vi "Teleop.vi"(10 "Match Info":T1={"Autonomous Elapsed Seconds"=0.0, "TeleOp Elapsed Seconds"=78.62, "Disabled Elapsed Seconds"=2.155, "Visited Autonomous"=FALSE, "Visited TeleOp"=TRUE, "Visited Disabled"=TRUE, "Autonomous Settings"={"Autonomous Style"=enum."Independent", "VI Refnum"=refnum}}, 11 "Call Context":T2=enum."Execute") -> ()   [LabVIEW 2017]
doc: "This VI is called for each enabled TeleOp packet received from the DS. It is typically used to read from joysticks and other inputs and update I/O or setpoints for timed control loops. It should complete and return within 20 milliseconds or risk missing DS packets."
uses:
  <vilib>/Rock Robotics/WPI/DriverStation/WPI_DriverStationDerivedRobotMode.ctl
  <vilib>/Rock Robotics/WPI/DriverStation/WPI_DriverStationMatch Info.ctl
  <vilib>/Rock Robotics/WPI/Utilities/WPI_GetSetVariantRefNum.vi
  <vilib>/Rock Robotics/Network Tables/NT Write Boolean Array.vi
  <vilib>/Rock Robotics/Network Tables/NT Write Numeric Array.vi
panel:
  in  "Right Setpoint":dbl=-1.0
  in  "Left Setpoint":dbl=-0.56
  in  "Bypass Joystick Sensitivity":bool
  in  "Turn Throtle (0 to +1)":dbl=1.0 min=0.0 max=1.0 step=0.1 format="%#_5g"
  in  "Speed Throtle (0 to +1)":dbl=0.5 min=0.0 max=1.0 step=0.1 format="%#_5g"
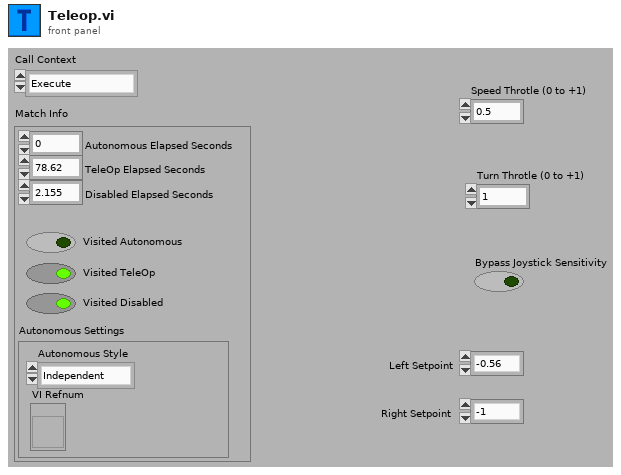
[diagram p1: front panel]
types:
  T1 = typedef "WPI_DriverStationMatch Info.ctl" = cluster{"Autonomous Elapsed Seconds":dbl, "TeleOp Elapsed Seconds":dbl, "Disabled Elapsed Seconds":dbl, "Visited Autonomous":bool, "Visited TeleOp":bool, "Visited Disabled":bool, "Autonomous Settings":cluster{"Autonomous Style":enum16{"Iterative", "Independent"}, "VI Refnum":refnum<vi>}}
  T2 = typedef "WPI_DriverStationDerivedRobotMode.ctl" = enum16{"Init", "Execute", "Stop"}
  T3 = typedef "WPI_JoystickDevRef.ctl" = cluster{"Device":T4}
  T4 = typedef "WPI_JoystickDeviceEnum.ctl" = enum16{"USB 0", "USB 1", "USB 2", "USB 3", "USB 4", "USB 5"}
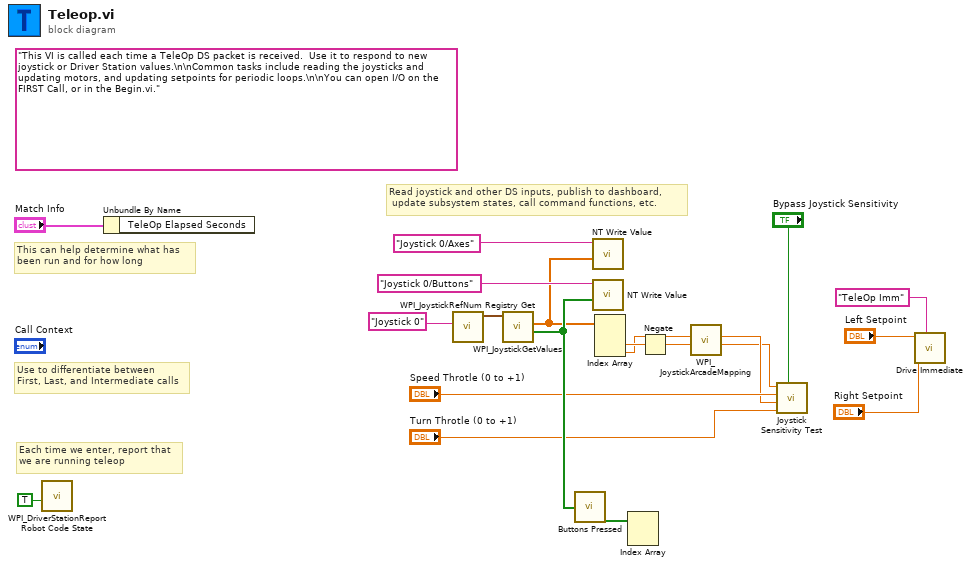
[diagram p0: block diagram]
diagram:
  (unwired) "This VI is called each time a TeleOp DS packet is received.  Use it to respond to new joystick or Driver Station values.\n\nCommon tasks include reading the joysticks and updating motors, and updating setpoints for periodic loops.\n\nYou can open I/O on the FIRST Call, or in the Begin.vi."
  # "Read joystick and other DS inputs, publish to dashboard,\n update subsystem states, call command functions, etc."
  # "Each time we enter, report that\nwe are running teleop"
  # "Use to differentiate between\nFirst, Last, and Intermediate calls"
  # "This can help determine what has\nbeen run and for how long"
  n1 = call <vilib>:"WPI_DriverStationReport Robot Code State.vi"("TeleOp"=TRUE ("Autonomous")) -> ()  [unwired: 10 in, 1 out]
  n2 = Unbundle By Name("Match Info") -> ()  [unwired: 1 out]
  n3 = call <vilib>:"WPI_JoystickRefNum Registry Get.vi"("refnum name"="Joystick 0") -> ("JoystickDevRef"=w17:T3)  [unwired: 1 in, 9 out]
  n4 = call <vilib>:"WPI_JoystickGetValues.vi"("JoystickDevRef"=w17) -> ("Buttons"=w12:bool[], "Axes"=w11:dbl[])  [unwired: 6 in, 3 out]
  n5 = call "Buttons Pressed.vi"("Button Values"=w12) -> ("Button Presses"=w15:bool[])
  n6 = call-poly <vilib>:"NT Write Value.vi"("Numeric Array"=w11, "Name"="Joystick 0/Axes") -> ()  [unwired: 9 in, 1 out]
  n7 = call-poly <vilib>:"NT Write Value.vi"("Boolean Array"=w12, "Name"="Joystick 0/Buttons") -> ()  [unwired: 9 in, 1 out]
  n8 = Index Array(array=w11) -> (element #2=w14:dbl, element #3=w5:dbl)  [unwired: 3 in, 1 out]
  n9 = Index Array(array=w15) -> ()  [unwired: 2 in, 2 out]
  n10 = Negate(x=w14) -> (-x=w6:dbl)
  n11 = call <vilib>:"WPI_JoystickArcadeMapping.vi"("Y axis value"=w6, "X axis value"=w5) -> ("Right Motor Value"=w3:dbl, "Left Motor Value"=w4:dbl)  [unwired: 8 in]
  n12 = call "Joystick Sensitivity Test.vi"("Bypass Joystick Sensitivity"="Bypass Joystick Sensitivity", "Turn Throtle (0 to +1)"="Turn Throtle (0 to +1)", "Turn Joystick Output (-1 to +1)"=w4, "Speed Throtle (0 to +1)"="Speed Throtle (0 to +1)", "Speed Joystick Output (-1 to +1)"=w3) -> ()  [unwired: 5 in, 2 out]
  n13 = call "Drive Immediate.vi"("Description"="TeleOp Imm", "Right Setpoint"="Right Setpoint", "Left Setpoint"="Left Setpoint") -> ()  [unwired: 8 in, 1 out]
